vi "WebDAV address (global).vi"(2 "Mode":enum16{"Read", "Write"}(ring), 3 "Network Drive Password":string, 8 "Network Drive IP":string) -> (0 "Password OUT":string, 5 "WebDAV Address":string)   [LabVIEW 2018]
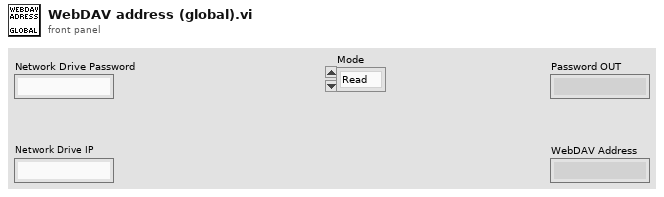
[diagram p1: front panel]
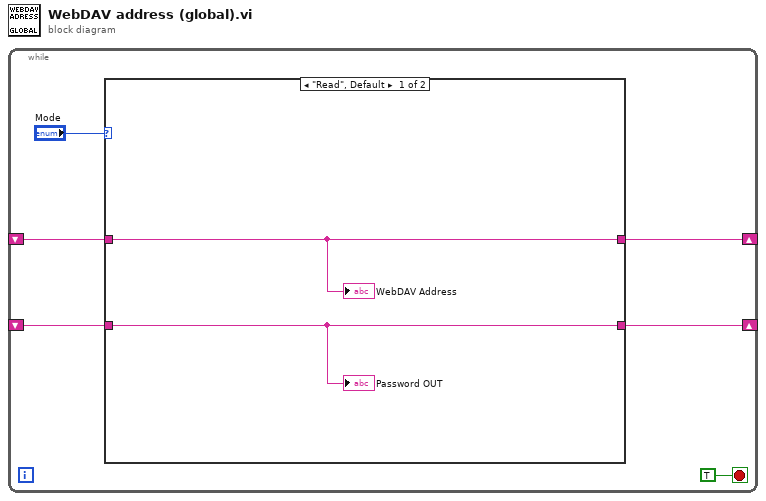
[diagram p0: block diagram]
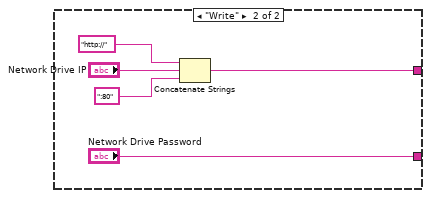
[diagram p2: hidden frame]
diagram:
  n1 = while {
    shift-right: [w4] -> _
    shift-left: _ -> [w3]
    shift-right: [w2] -> _
    shift-left: _ -> [w1]
    stop <- TRUE stop-if-true
    n2 = case shown="\"Read\", Default" "Mode" {
      tunnel: [w8 w10] -> w4
      tunnel: w3 -> [w8 _]
      tunnel: [w7 "Network Drive Password"] -> w2
      tunnel: w1 -> [w7 _]
      frame "Read", Default {
        "WebDAV Address" <- w8
        "Password OUT" <- w7
      }
      frame "Write" {
        n3 = Concatenate Strings("http://", "Network Drive IP", ":80") -> (w10:string)
      }
    }
  }
